vi "SwerveGlobals.vi"() -> ()   [LabVIEW 2018]
panel:
  in  "ReleaseCargo":bool
  in  "IR":dbl
  out "ErrorMessage":string
  out "LiftLevel":enum16{"Low", "Mid", "High"}(ring)
  in  "ArmOut":bool
  in  "ReleaseHatch":bool
  in  "ZeroGyro":bool
  in  "VisionAlign":bool
  in  "DriveMode":enum16{"Swerve", "Ackerman"}(ring)
  in  "Gyro":dbl
  in  "ZAxis":dbl
  in  "YAxis":dbl
  in  "XAxis":dbl
  # "Code:"
  # "Pilot:"
  # "Copilot:"
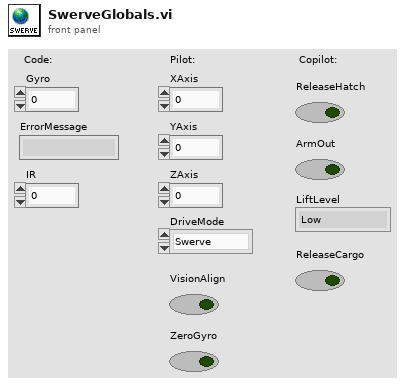
[diagram p1: front panel]
diagram:
